vi "MP-285 GetSet Speed.vi"(3 "error in (no error)":errorcluster, 4 "Input: Speed in microns/sec":i32, 5 "VISA resource name":refnum<visa-resource-name>) -> (0 "error out":errorcluster, 1 "Output: Speed in microns/sec":u32, 2 "VISA resource name 2":refnum<visa-resource-name>)   [LabVIEW 2010]
panel:
  out "Word to MP-285":string
  out "Serial Read":string
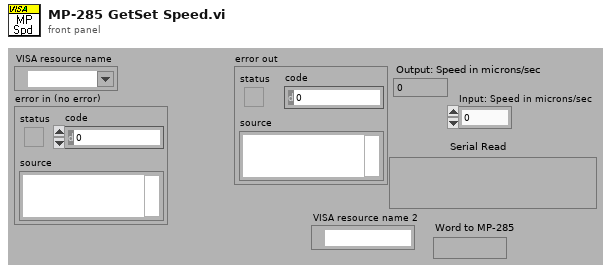
[diagram p1: front panel]
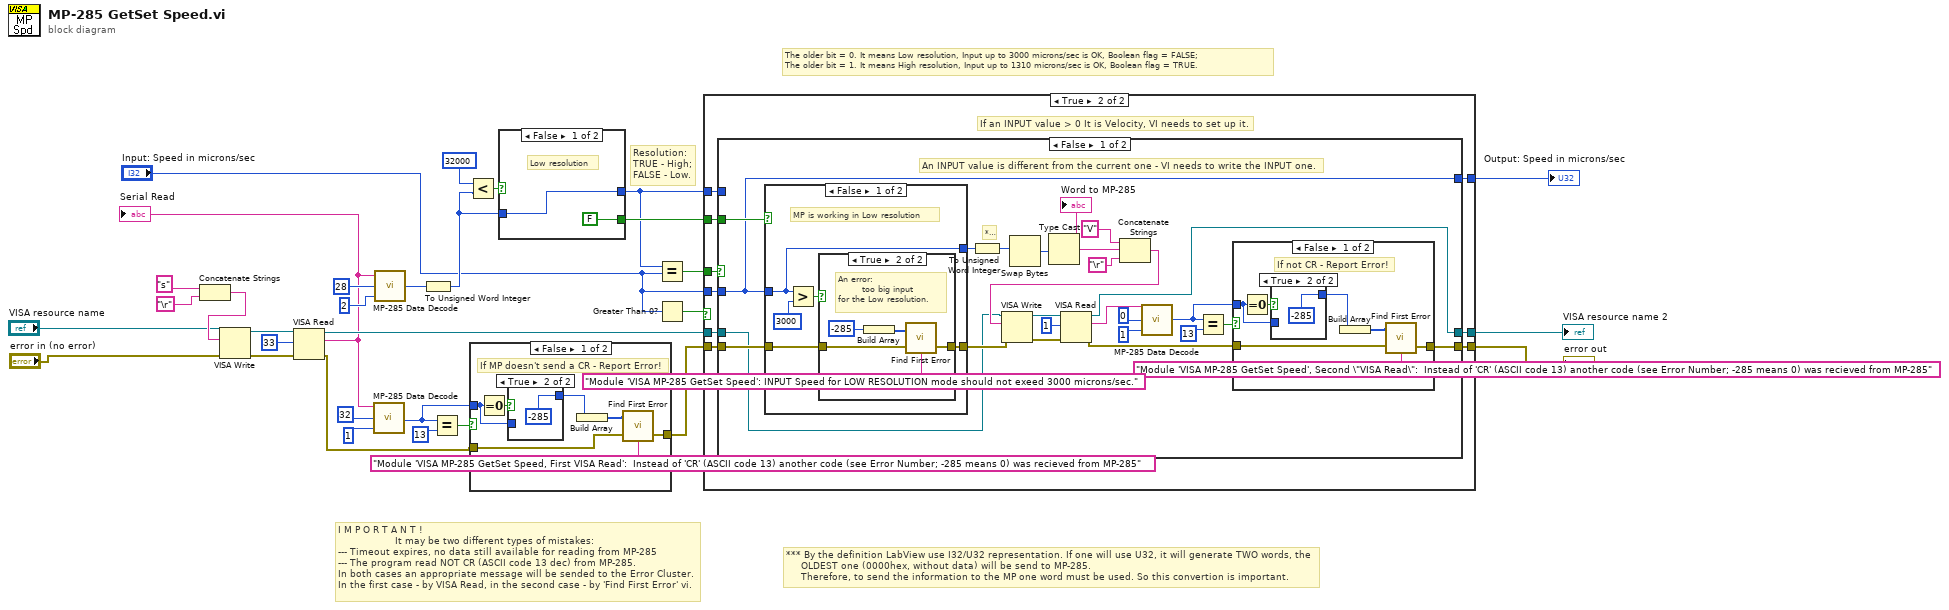
[diagram p0: block diagram]
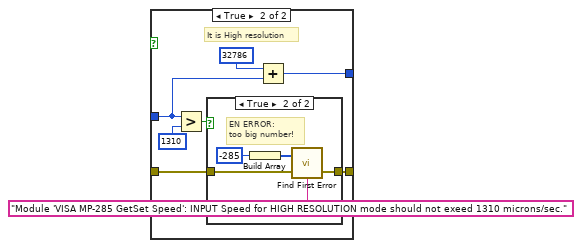
[diagram p6: hidden frame]
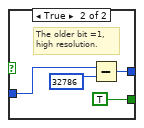
[diagram p9: hidden frame]
diagram:
  # "*** By the definition LabView use I32/U32 representation. If one will use U32, it will generate TWO words, the \n     OLDEST one (0000hex, without data) will be send to MP-285. \n     Therefore, to send the information to the MP one word must be used. So this convertion is important."
  # "The older bit = 0. It means Low resolution, Input up to 3000 microns/sec is OK, Boolean flag = FALSE;\nThe older bit = 1. It means High resolution, Input up to 1310 microns/sec is OK, Boolean flag = TRUE."
  # "Resolution:\nTRUE - High;\nFALSE - Low."
  # "I M P O R T A N T !\n                   It may be two different types of mistakes: \n--- Timeout expires, no data still available for reading from MP-285\n--- The program read NOT CR (ASCII code 13 dec) from MP-285.\nIn both cases an appropriate message will be sended to the Error Cluster.\nIn the first case - by VISA Read, in the second case - by 'Find First Error' vi."
  n1 = Concatenate Strings("s", "\r") -> (w29:string)
  n2 = VISA Write(VISA resource name="VISA resource name", write buffer=w29, error in (no error)="error in (no error)") -> (VISA resource name out=w28:refnum<visa-resource-name>, error out=w27:errorcluster)  [unwired: 1 out]
  n3 = VISA Read(VISA resource name=w28, byte count=33, error in (no error)=w27) -> (VISA resource name out=w22:refnum<visa-resource-name>, read buffer=w5:string, error out=w17:errorcluster)  [unwired: 1 out]
  "Serial Read" <- w5
  n4 = call "MP-285 Data Decode.vi"("Input: lenght"=1, "Input: offset"=32, "Input: Data string"=w5) -> ("Output: Decoded Data"=w23:i32)
  n5 = call "MP-285 Data Decode.vi"("Input: lenght"=2 ("length"), "Input: offset"=28 ("offset (0)"), "Input: Data string"=w5) -> ("Output: Decoded Data"=w19:i32)
  n6 = To Unsigned Word Integer(number=w19) -> (unsigned 16bit integer=w18:u16)
  n7 = Equal?(x=w23, y=13) -> (x = y?=w24:bool)
  n8 = Less?(x=32000, y=w18) -> (x < y?=w21:bool)
  n9 = case shown="False" w24 {
    tunnel: [w38 w41] -> w16
    tunnel: w23 -> [w34 _]
    tunnel: w17 -> [w32 w41]
    frame False {
      # "If MP doesn't send a CR - Report Error!"
      n10 = Equal To 0?(x=w34) -> (x = 0?=w35:bool)
      n11 = case shown="True" w35 {
        tunnel: w34 -> [w39 _]
        tunnel: [w39 -285] -> w33
        frame False {
        }
        frame True {
        }
      }
      n12 = Build Array(w33) -> (w36:i32[])
      n13 = call <vilib>:"Find First Error.vi"("error in (no error)"=w32, "source messages"="Module 'VISA MP-285 GetSet Speed, First VISA Read':  Instead of 'CR' (ASCII code 13) another code (see Error Number; -285 means 0) was recieved from MP-285", "error codes"=w36) -> ("error out"=w38:errorcluster)  [unwired: 2 out]
    }
    frame True {
      # "TRUE: CR was received - NO Errors"
    }
  }
  n14 = case shown="False" w21 {
    tunnel: [w43 w47] -> w11
    tunnel: w18 -> [w43 w45]
    tunnel: [FALSE TRUE] -> w14
    frame False {
      # "Low resolution"
    }
    frame True {
      # "The older bit =1, \nhigh resolution."
      n15 = Subtract(x=w45, y=32786) -> (x-y=w47:i32)
    }
  }
  n16 = Equal?(x=w11, y="Input: Speed in microns/sec") -> (x = y?=w15:bool)
  n17 = Greater Than 0?(x="Input: Speed in microns/sec") -> (x > 0?=w13:bool)
  n18 = case shown="True" w13 {
    tunnel: w22 -> [w50 w59]
    tunnel: w16 -> [w49 w58]
    tunnel: w15 -> [_ w57]
    tunnel: [w50 w56] -> w2
    tunnel: [w49 w55] -> w1
    tunnel: w14 -> [_ w54]
    tunnel: "Input: Speed in microns/sec" -> [_ w53]
    tunnel: w11 -> [w48 w52]
    tunnel: [w48 w51] -> w10
    frame False {
      # "If an INPUT value <=0 there is nothing to write, just output the current Velocity."
    }
    frame True {
      # "If an INPUT value > 0 It is Velocity, VI needs to set up it."
      n19 = case shown="False" w57 {
        tunnel: w58 -> [w82 w120]
        tunnel: w59 -> [w75 w119]
        tunnel: [w69 w120] -> w55
        tunnel: [w62 w119] -> w56
        tunnel: w54 -> [w83 _]
        tunnel: w53 -> [w64 _]
        tunnel: w52 -> [_ w118]
        tunnel: [w64 w118] -> w51
        frame False {
          # "***"
          # "An INPUT value is different from the current one - VI needs to write the INPUT one."
          n20 = case shown="False" w83 {
            tunnel: w64 -> [w98 w108]
            tunnel: w82 -> [w95 w109]
            tunnel: [w98 w106] -> w66
            tunnel: [w94 w105] -> w76
            frame False {
              # "MP is working in Low resolution"
              n21 = Greater?(x=w98, y=3000) -> (0:w96:bool)
              n22 = case shown="True" w96 {
                tunnel: w95 -> [w99 w104]
                tunnel: [w99 w103] -> w94
                frame False {
                  # "An INPUT is\nin range."
                }
                frame True {
                  # "An error:\n        too big input\nfor the Low resolution."
                  n23 = Build Array(-285) -> (w101:i32[])
                  n24 = call <vilib>:"Find First Error.vi"("error in (no error)"=w104, "source messages"="Module 'VISA MP-285 GetSet Speed': INPUT Speed for LOW RESOLUTION mode should not exeed 3000 microns/sec.", "error codes"=w101) -> ("error out"=w103:errorcluster)  [unwired: 2 out]
                }
              }
            }
            frame True {
              # "It is High resolution"
              n25 = Greater?(x=w108, y=1310) -> (0:w110:bool)
              n26 = case shown="True" w110 {
                tunnel: w109 -> [w112 w116]
                tunnel: [w112 w117] -> w105
                frame False {
                  # "Input correct, \nWe can write."
                }
                frame True {
                  # "EN ERROR:\ntoo big number!"
                  n27 = Build Array(-285) -> (w114:i32[])
                  n28 = call <vilib>:"Find First Error.vi"("error in (no error)"=w116, "source messages"="Module 'VISA MP-285 GetSet Speed': INPUT Speed for HIGH RESOLUTION mode should not exeed 1310 microns/sec.", "error codes"=w114) -> ("error out"=w117:errorcluster)  [unwired: 2 out]
                }
              }
              n29 = Add(x=32786, y=w108) -> (x+y=w106:i32)
            }
          }
          n30 = To Unsigned Word Integer(number=w66) -> (unsigned 16bit integer=w65:u16)
          n31 = Swap Bytes(anything=w65) -> (byte swapped=w68:u16)
          n32 = Type Cast(x=w68) -> (*(type *) &x=w67:string)  [unwired: 1 out]
          "Word to MP-285" <- w67
          n33 = Concatenate Strings("V", w67, "\r") -> (w80:string)
          n34 = VISA Write(VISA resource name=w75, write buffer=w80, error in (no error)=w76) -> (VISA resource name out=w79:refnum<visa-resource-name>, error out=w78:errorcluster)  [unwired: 1 out]
          n35 = VISA Read(VISA resource name=w79, byte count=1, error in (no error)=w78) -> (VISA resource name out=w62:refnum<visa-resource-name>, read buffer=w63:string, error out=w70:errorcluster)  [unwired: 1 out]
          n36 = call "MP-285 Data Decode.vi"("Input: lenght"=1, "Input: offset"=0, "Input: Data string"=w63) -> ("Output: Decoded Data"=w71:i32)
          n37 = Equal?(x=w71, y=13) -> (x = y?=w72:bool)
          n38 = case shown="False" w72 {
            tunnel: [w90 w93] -> w69
            tunnel: w71 -> [w86 _]
            tunnel: w70 -> [w84 w93]
            frame False {
              # "If not CR - Report Error!"
              n39 = Equal To 0?(x=w86) -> (x = 0?=w87:bool)
              n40 = case shown="True" w87 {
                tunnel: w86 -> [w91 _]
                tunnel: [w91 -285] -> w85
                frame False {
                }
                frame True {
                }
              }
              n41 = Build Array(w85) -> (w88:i32[])
              n42 = call <vilib>:"Find First Error.vi"("error in (no error)"=w84, "source messages"="Module 'VISA MP-285 GetSet Speed', Second \"VISA Read\":  Instead of 'CR' (ASCII code 13) another code (see Error Number; -285 means 0) was recieved from MP-285", "error codes"=w88) -> ("error out"=w90:errorcluster)  [unwired: 2 out]
            }
            frame True {
              # "TRUE CR was received - NO Errors"
            }
          }
        }
        frame True {
          # "An INPUT value is the same, as current one --> Nothing to do!"
        }
      }
    }
  }
  "Output: Speed in microns/sec" <- w10
  "VISA resource name 2" <- w2
  "error out" <- w1
